vi "Write Teller.vi"(10 "Teller":refnum<class "Teller.lvclass">, 11 "Msg Input in":refnum<class "Msg Input.lvclass">) -> (3 "Msg Input out":refnum<class "Msg Input.lvclass">)   [LabVIEW 2020, in "jettl.lvlib" / "Msg Input.lvclass"]
uses:
  Msg Input.lvclass
  Teller/Teller.lvclass
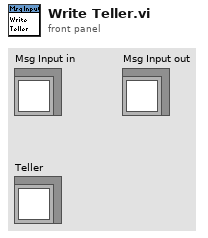
[diagram p1: front panel]
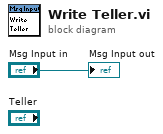
[diagram p0: block diagram]
diagram:
  "Msg Input out" <- "Msg Input in"
